vi "Memory.Pointer.Allocate.vi"   [LabVIEW 2016, in "LabVIEW Memory Manager.lvlib" / "Memory.Pointer.lvclass"]
uses:
  Memory.Pointer.lvclass
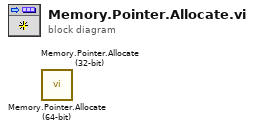
[diagram p0: block diagram]
diagram:
  n1 = call "Memory.Pointer.Allocate (64-bit).vi"() -> ()  [unwired: 10 in, 2 out]
  n2 = call "Memory.Pointer.Allocate (32-bit).vi"() -> ()  [unwired: 10 in, 2 out]
